vi "SCLN_ShutdownMessage.vi"(0 "Server Number":i32 min=0 max=50) -> ()   [LabVIEW 2015]
uses:
  SCLN_RW_Select.ctl
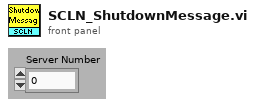
[diagram p1: front panel]
types:
  T1 = typedef "SCLN_RW_Select.ctl" = enum16{"Read", "Write"}
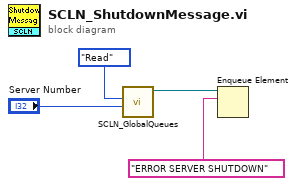
[diagram p0: block diagram]
diagram:
  n1 = call "SCLN_GlobalQueues.vi"("Element"="Server Number", "Operation"=SCLN_RW_Select."Read" ("GBL_RW")) -> ("Read QueueID"=w2:refnum<queue>)  [unwired: 6 in, 1 out]
  n2 = Enqueue Element(queue=w2, element="ERROR SERVER SHUTDOWN") -> ()  [unwired: 2 in, 3 out]
